vi "Call Check and Download Bitfile.vi"(8 "error in":errorcluster, 9 "Target IP Address":string, 10 "Bitfile Path":path, 11 "Slave Ref":string) -> (0 "error out":errorcluster)   [LabVIEW 2019, in "SEECD System Explorer.lvlib"]
uses:
  SEECD System Explorer.lvlib
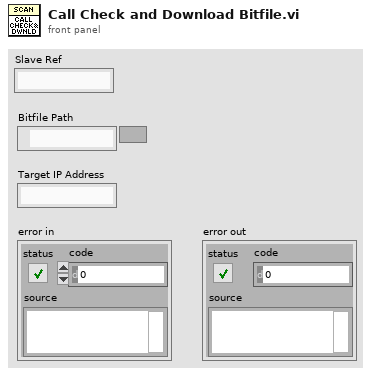
[diagram p1: front panel]
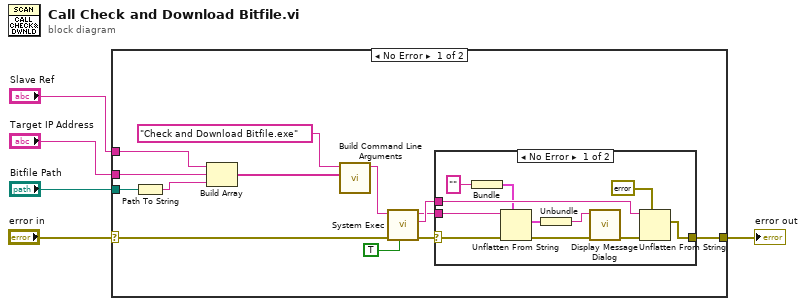
[diagram p0: block diagram]
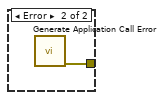
[diagram p2: hidden frame]
diagram:
  n1 = case shown="No Error" "error in" {
    selector: "error in" -> [w18 w31]
    tunnel: [w8 w31] -> w1
    tunnel: "Slave Ref" -> [w15 _]
    tunnel: "Target IP Address" -> [w14 _]
    tunnel: "Bitfile Path" -> [w16 _]
    frame No Error {
      n2 = Path To String(path=w16) -> (string=w13:string)
      n3 = Build Array(w15, w14, w13) -> (w12:string[])
      n4 = call "Build Command Line Arguments.vi"("Arguments"=w12, "Executable File Name"="Check and Download Bitfile.exe" ("name or relative path")) -> ("Command Line"=w10:string)  [unwired: 9 in]
      n5 = call <vilib>:"System Exec.vi"("run minimized? (F)"=TRUE, "error in (no error)"=w18, "command line"=w10) -> ("error out"=w9:errorcluster, "standard error"=w7:string, "standard output"=w6:string)  [unwired: 5 in, 1 out]
      n6 = case shown="No Error" w9 {
        selector: w9 -> [w25 _]
        tunnel: [w28 w30] -> w8
        tunnel: w7 -> [w27 _]
        tunnel: w6 -> [w22 _]
        frame No Error {
          n7 = Bundle("") -> (w23:cluster{string})  [unwired: 1 in]
          n8 = Unflatten From String(type=w23, binary string=w22, error in (no error)=w25) -> (value=w20:cluster{string}, error out=w24:errorcluster)  [unwired: 2 in, 1 out]
          n9 = Unbundle(w20) -> (w19:string)
          n10 = call "Display Message Dialog.vi"("error in"=w24, "Message to display"=w19) -> ("error out"=w26:errorcluster)  [unwired: 9 in]
          n11 = Unflatten From String(type=errorcluster {"status"=FALSE, "code"=0, "source"=""} ("error in (no error)"), binary string=w27, error in (no error)=w26) -> (value=w28:errorcluster)  [unwired: 2 in, 2 out]
        }
        frame Error {
          n12 = call "Generate Application Call Error.vi"() -> ("error out"=w30:errorcluster)  [unwired: 11 in]
        }
      }
    }
    frame Error {
    }
  }
  "error out" <- w1
